vi "Launch Updater.vi"(8 "error in (no error)":errorcluster, 11 "Config Monitor Module in":refnum<class "Config Monitor Module.lvclass">) -> (0 "error out":errorcluster, 3 "Config Monitor Module out":refnum<class "Config Monitor Module.lvclass">)   [LabVIEW 2020, in "VolatusGUI.lvlib" / "Config Monitor Module.lvclass"]
uses:
  Config Monitor Module.lvclass
  Config Monitor Module.lvclass/Config Monitor Module.ctl
  Git Updater Module/Git Updater Module.lvclass
  Module/Module.lvclass
  VolatusConfig/VolatusConfigElement/VolatusConfigElement.lvclass
  C:/dev/lv20CE/relink/lv-volatus/Volatus/Module/Module.lvclass
  C:/dev/lv20CE/relink/lv-volatus/Volatus/Git Updater Module/Git Updater Module.lvclass
  C:/dev/lv20CE/relink/lv-volatus/Volatus/Config Alert Module/Config Monitor Module.lvclass
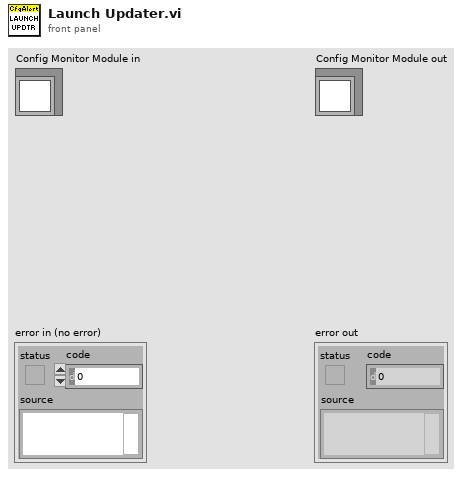
[diagram p1: front panel]
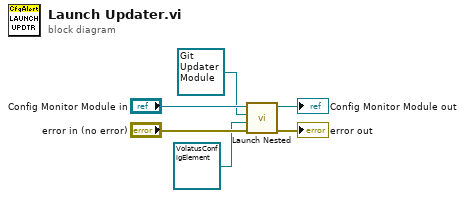
[diagram p0: block diagram]
diagram:
  n1 = call "Launch Nested.vi"("error in (no error)"="error in (no error)", "Config Element"=refnum<class "VolatusConfigElement.lvclass"> refnum, "Nested Module"=refnum<class "Git Updater Module.lvclass"> refnum ("VolatusGUI:Config Updater Module.lvclass"), "Parent in"="Config Monitor Module in") -> ("error out"=→"error out":errorcluster, "Parent out"=→"Config Monitor Module out":refnum<class "Config Monitor Module.lvclass">)  [unwired: 5 in, 1 out]
